vi "File Name.vi"(11 "string":string=" Test.txt") -> (3 "String":string)   [LabVIEW 2020]
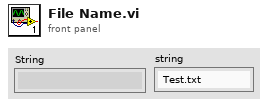
[diagram p1: front panel]
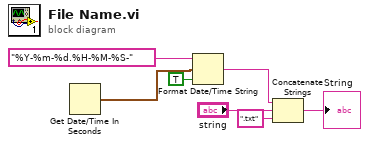
[diagram p0: block diagram]
diagram:
  n1 = Get Date/Time In Seconds() -> (seconds since 1Jan1904=w3:timestamp)
  n2 = Format Date/Time String(time format string (%c)="%Y-%m-%d.%H-%M-%S-", seconds (now)=w3, UTC format=TRUE) -> (date/time string=w5:string)
  n3 = Concatenate Strings(w5, "string", ".txt" ("string")) -> (→"String":string)
